vi "Update Map Color.vi"(8 "error in (no error)":errorcluster, 10 "Old Color Table":T1={"Occupied Color"={"Value"=0, "Color"=0}, "Free Color"={"Value"=205, "Color"=16777215}, "Unknown Color"={"Value"=254, "Color"=13421772}}, 11 "Map Model in":refnum<class "Map Model.lvclass">) -> (0 "error out":errorcluster, 3 "Map Model out":refnum<class "Map Model.lvclass">)   [LabVIEW 2020, in "Map Model.lvlib" / "Map Model.lvclass"]
uses:
  Map Model.lvclass
  Map Model.lvclass/Map Model.ctl
  <vilib>/picture/picture.llb/Draw 4-Bit Pixmap.vi
panel:
  # "NOTICE -- YOU MUST LEAVE THIS NOTICE IN PLACE.\n\nCopyright (c) 2017, LIANG LIU Shawn.Liu.cn@gmail.com\nAll rights reserved.\n\nRedistribution and use in source and binary forms, with or without modification, are permitted provided that the following conditions are met:\n-Redistributions of source code must retain the above copyright notice, this list of conditions and the following disclaimer.\n-Redistributions in binary form must reproduce the above copyright notice, this list of conditions and the following disclaimer in the documentation and/or other materials provided with the distribution.\n-Neither the name of the eLp nor the names of its contributors may be used to endorse or promote products derived from this software without specific prior written permission.\n\nTHIS SOFTWARE IS PROVIDED BY THE COPYRIGHT HOLDERS AND CONTRIBUTORS \"AS IS\" AND ANY EXPRESS OR IMPLIED WARRANTIES, INCLUDING, BUT NOT LIMITED TO, THE IMPLIED WARRANTIES OF MERCHANTABILITY AND FITNESS FOR A PARTICULAR PURPOSE ARE DISCLAIMED. IN NO EVENT SHALL THE COPYRIGHT HOLDER OR CONTRIBUTORS BE LIABLE FOR ANY DIRECT, INDIRECT, INCIDENTAL, SPECIAL, EXEMPLARY, OR CONSEQUENTIAL DAMAGES (INCLUDING, BUT NOT LIMITED TO, PROCUREMENT OF SUBSTITUTE GOODS OR SERVICES; LOSS OF USE, DATA, OR PROFITS; OR BUSINESS INTERRUPTION) HOWEVER CAUSED AND ON ANY THEORY OF LIABILITY, WHETHER IN CONTRACT, STRICT LIABILITY, OR TORT (INCLUDING NEGLIGENCE OR OTHERWISE) ARISING IN ANY WAY OUT OF THE USE OF THIS SOFTWARE, EVEN IF ADVISED OF THE POSSIBILITY OF SUCH DAMAGE."
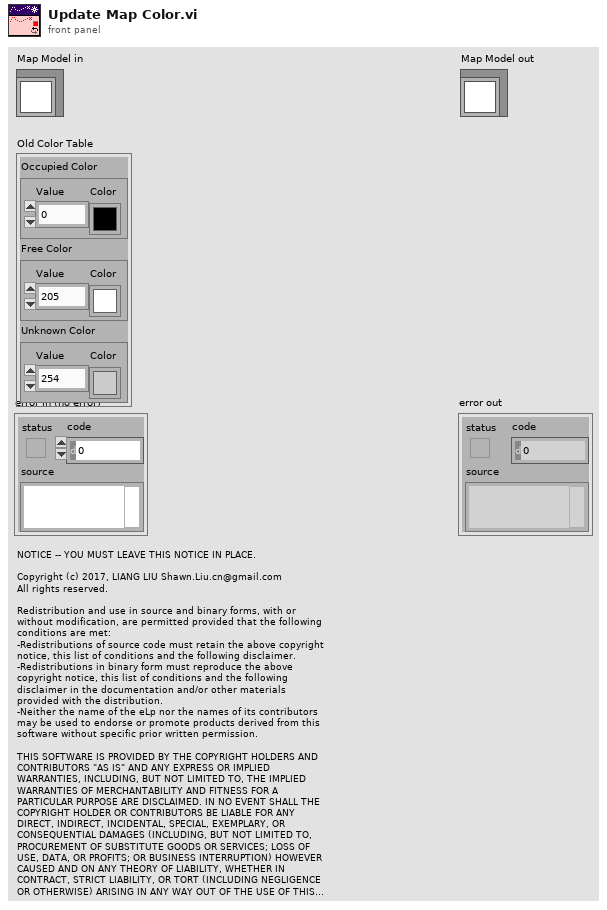
[diagram p1: front panel]
types:
  T1 = cluster{"Occupied Color":cluster{"Value":u8, "Color":u32}, "Free Color":cluster{"Value":u8, "Color":u32}, "Unknown Color":cluster{"Value":u8, "Color":u32}}
  T2 = typedef "imagedata.ctl" = cluster{"image type":i32, "image depth":i32, "image":u8[], "mask":u8[], "colors":u32[], "Rectangle":cluster{"left":i16, "top":i16, "right":i16, "bottom":i16}}
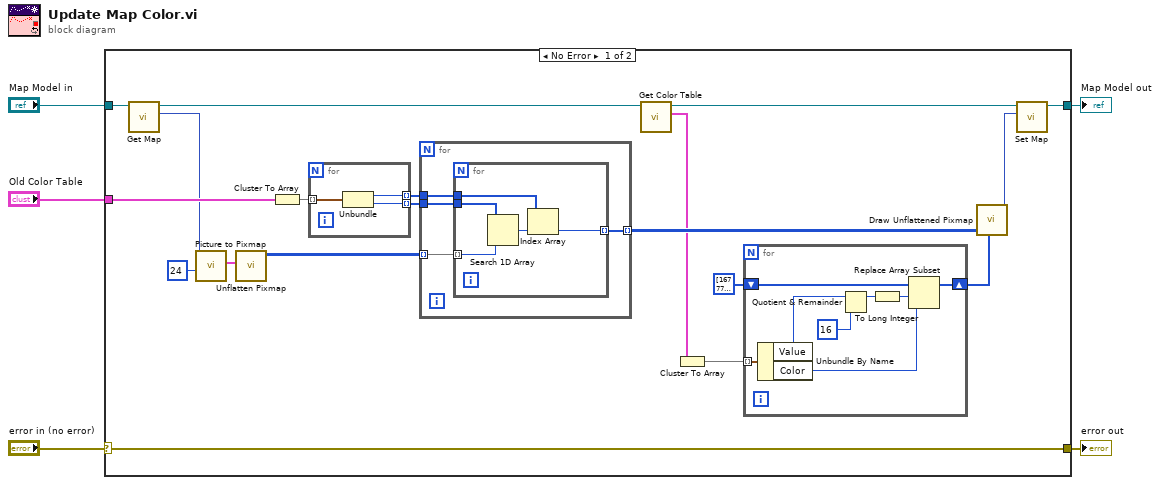
[diagram p0: block diagram]
diagram:
  n1 = case shown="No Error" "error in (no error)" {
    selector: "error in (no error)" -> [w22 w46]
    tunnel: "Map Model in" -> [w24 w45]
    tunnel: [w23 w45] -> w4
    tunnel: "Old Color Table" -> [w21 _]
    tunnel: [w22 w46] -> w1
    frame No Error {
      n2 = call "Get Map.vi"("Map Model in"=w24) -> ("Map"=w9:picture, "Map Model out"=w20:refnum<class "Map Model.lvclass">)  [unwired: 9 in]
      n3 = call <vilib>:"Picture to Pixmap.vi"("depth"=24, "picture"=w9) -> ("image data"=w19:T2)  [unwired: 8 in, 1 out]
      n4 = call <vilib>:"Unflatten Pixmap.vi"("image data"=w19) -> ("24-bit pixmap"=w16:u32[][])  [unwired: 4 in, 6 out]
      n5 = Cluster To Array(cluster=w21) -> (array=w8:cluster{"Value":u8, "Color":u32}[])
      n6 = for {
        tunnel: w8 -> [w35] mode=indexing
        tunnel: [w34] -> w15 mode=indexing
        tunnel: [w33] -> w17 mode=indexing
        n7 = Unbundle(w35) -> ("Value"=w34:u8, "Color"=w33:u32)
      }
      n8 = for {
        tunnel: w16 -> [w39] mode=indexing
        tunnel: [w38] -> w13 mode=indexing
        tunnel: w17 -> [w37]
        tunnel: w15 -> [w36]
        n9 = for {
          tunnel: w39 -> [w41] mode=indexing
          tunnel: [w40] -> w38 mode=indexing
          tunnel: w37 -> [w42]
          tunnel: w36 -> [w44]
          n10 = Search 1D Array(1D array=w42, element=w41) -> (index of element=w43:i32)  [unwired: 1 in]
          n11 = Index Array(array=w44, index=w43) -> (element=w40:u8)
        }
      }
      n12 = call "Get Color Table.vi"("Map Model in"=w20) -> ("Color Table"=w7:T1, "Map Model out"=w12:refnum<class "Map Model.lvclass">)  [unwired: 9 in]
      n13 = Cluster To Array(cluster=w7) -> (array=w10:cluster{"Value":u8, "Color":u32}[])
      n14 = for {
        shift-right: [w31] -> w6
        shift-left: u32[] [16777215, 16776960, 128, 16711680, 16711935, 8388736, 255, 65535, 65280, 32768, 8388608, 8421376, 12632256, 8421504, 32896, 0] ("color table") -> [w32]
        tunnel: w10 -> [w30] mode=indexing
        n15 = Unbundle By Name(w30) -> ("Value"=w29:u8, "Color"=w27:u32)
        n16 = Quotient & Remainder(x=w29, y=u8 16) -> (x-y*floor(x/y)=w28:u8)  [unwired: 1 out]
        n17 = To Long Integer(number=w28) -> (32bit integer=w26:i32)
        n18 = Replace Array Subset(array=w32, new element=w27, index=w26) -> (w31:u32[])
      }
      n19 = call-poly <vilib>:"Draw Unflattened Pixmap.vi"("data"=w13, "color table"=w6) -> ("new picture"=w11:picture)  [unwired: 7 in]
      n20 = call "Set Map.vi"("Map"=w11, "Map Model in"=w12) -> ("Map Model out"=w23:refnum<class "Map Model.lvclass">)  [unwired: 9 in]
    }
    frame Error {
    }
  }
  "error out" <- w1
  "Map Model out" <- w4
